vi "lvstyx_usb_search.vi"(8 "error in (no error)":errorcluster, 9 "pid":u16=2048, 10 "vid":u16=2048, 11 "conn ptr":u32) -> (0 "error out":errorcluster, 2 "found?":bool, 3 "dup conn ptr":u32)   [LabVIEW 2010, in "lib1299.lvlib"]
uses:
  lib1299.lvlib
  cstyx/win32/cstyx.dll
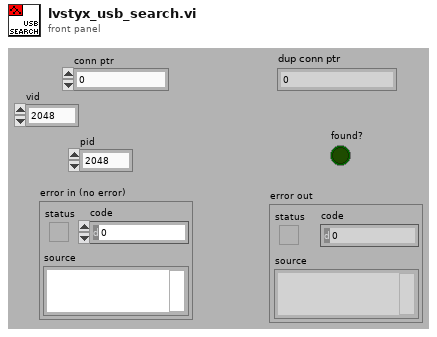
[diagram p1: front panel]
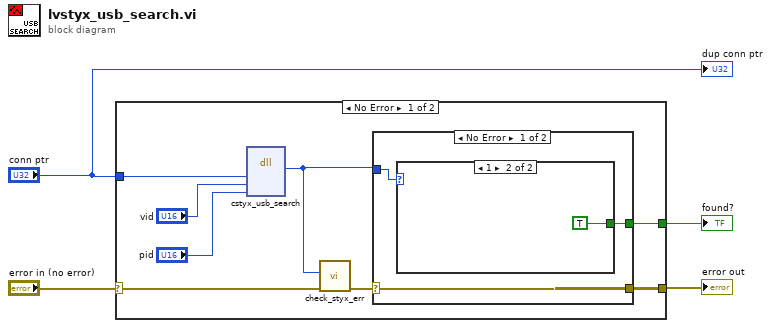
[diagram p0: block diagram]
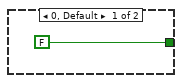
[diagram p2: hidden frame]
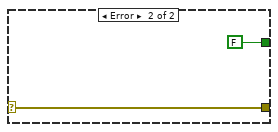
[diagram p3: hidden frame]
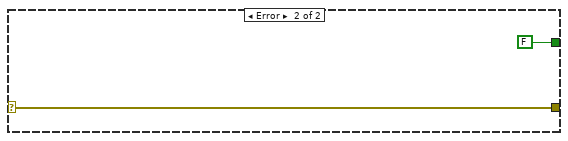
[diagram p4: hidden frame]
diagram:
  n1 = case shown="No Error" "error in (no error)" {
    selector: "error in (no error)" -> [w11 w21]
    tunnel: "conn ptr" -> [w12 _]
    tunnel: [w5 w21] -> w4
    tunnel: [w6 FALSE ("found?")] -> w1
    frame No Error {
      n2 = dll-call lib="C:/work/ads1299evm/lib_1299/Styx/cstyx/win32/cstyx.dll" fn="cstyx_usb_search"("conn"=w12, "vid"="vid", "pid"="pid") -> ("result"=w7:i32)  [unwired: 6 in, 2 out]
      n3 = call "check_styx_err.vi"("error in (no error)"=w11, "return val"=w7) -> ("error out"=w8:errorcluster)  [unwired: 9 in]
      n4 = case shown="No Error" w8 {
        selector: w8 -> [w13 w18]
        tunnel: w7 -> [w15 _]
        tunnel: [w14 FALSE ("found?")] -> w6
        tunnel: [w13 w18] -> w5
        frame No Error {
          n5 = case shown="1" w15 {
            tunnel: [FALSE ("found?") TRUE ("found?")] -> w14
            frame 0, Default {
            }
            frame 1 {
            }
          }
        }
        frame Error {
        }
      }
    }
    frame Error {
    }
  }
  "error out" <- w4
  "found?" <- w1
  "dup conn ptr" <- "conn ptr"
